vi "DetermineStateOfBoat-OLD.vi"() -> (2 "TimeSpentInCurrentState (s)":dbl, 3 "StateOfBoat":T1)   [LabVIEW 2013]
doc: "Eric Schneider and Bonnie Ishiguro\n1/24/14\n\nDetermineStateOfBoat should take in data from the forebrain about the plan of the boat (tacking, jibing, straight, distance to waypoint) as well as robot variables (heading, desired heading, wind speed, etc.) and makes a judgement about the qualitative state of the boat.\n\nThese qualitative states are intended to represent several different rules of sail/rudder control - which rules the sail/rudder should follow should change in each state. The set of current states is by no means set in stone, but should be tweaked with sailing advice so that in the end we have a handful of sailing states that each has a different control scheme for sail/rudder."
uses:
  Data/TypeDefs/Sailing State of Boat.ctl
panel:
  in  "Forebrain Maneuver\nCommand (PLACEHOLDER)":enum16{"No Maneuver", "Tack Now", "Jibe Now"}(ring)
  in  "MaxStayForce":dbl
  in  "WindSpeed (m/s)":dbl
  in  "HindbrainEmergencySailOverrideOn":bool
  in  "BoatSpeed (m/s)":dbl
  in  "RelativeWind (0-180)":dbl
  in  "DesiredHeading (0-360)":dbl
  in  "RobotHeading (0-360)":dbl
  in  "DistanceToNextWaypoint (m)":dbl=10.0
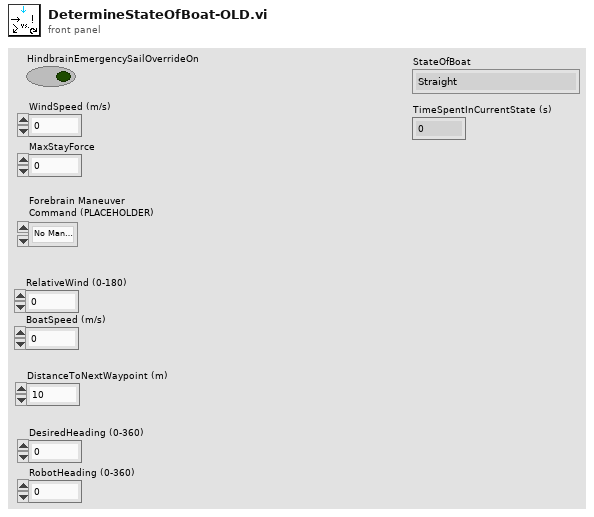
[diagram p1: front panel]
types:
  T1 = typedef "Sailing State of Boat.ctl" = enum16{"Straight", "Turning", "Approach Maneuver", "Cross Wind (Tack)", "Cross Wind (Jibe)", "Stuck in irons", "Turtle Mode"}
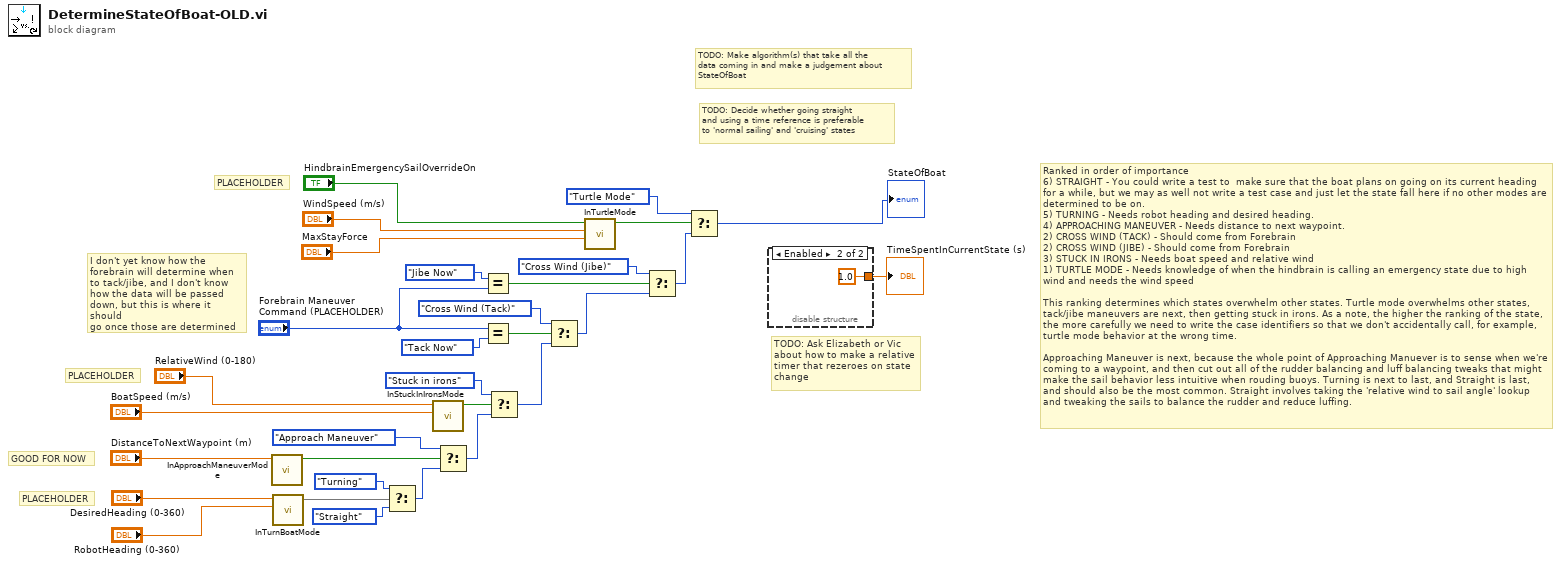
[diagram p0: block diagram]
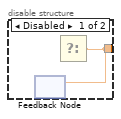
[diagram p2: hidden frame]
diagram:
  # "PLACEHOLDER"
  # "PLACEHOLDER"
  # "GOOD FOR NOW"
  # "PLACEHOLDER"
  # "I don't yet know how the\nforebrain will determine when\nto tack/jibe, and I don't know\nhow the data will be passed\ndown, but this is where it should\ngo once those are determined"
  # "Ranked in order of importance\n6) STRAIGHT - You could write a test to  make sure that the boat plans on going on its current heading for a while, but we may as well not write a test case and just let the state fall here if no other modes are determined to be on.\n5) TURNING - Needs robot heading and desired heading.\n4) APPROACHING MANEUVER - Needs distance to next waypoint.\n2) CROSS WIND (TACK) - Should come from Forebrain\n2) CROSS WIND (JIBE) - Should come from Forebrain\n3) STUCK IN IRONS - Needs boat speed and relative wind\n1) TURTLE MODE - Needs knowledge of when the hindbrain is calling an emergency state due to high wind and needs the wind speed\n\nThis ranking determines which states overwhelm other states. Turtle mode overwhelms other states, tack/jibe maneuvers are next, then getting stuck in irons. As a note, the higher the ranking of the state, the more carefully we need to write the case identifiers so that we don't accidentally call, for example, turtle mode behavior at the wrong time.\n\nApproaching Maneuver is next, because the whole point of Approaching Manuever is to sense when we're coming to a waypoint, and then cut out all of the rudder balancing and luff balancing tweaks that might make the sail behavior less intuitive when rouding buoys. Turning is next to last, and Straight is last, and should also be the most common. Straight involves taking the 'relative wind to sail angle' lookup and tweaking the sails to balance the rudder and reduce luffing."
  # "TODO: Ask Elizabeth or Vic about how to make a relative timer that rezeroes on state change"
  # "TODO: Decide whether going straight\nand using a time reference is preferable\nto 'normal sailing' and 'cruising' states"
  # "TODO: Make algorithm(s) that take all the\ndata coming in and make a judgement about\nStateOfBoat"
  n1 = call "InApproachManeuverMode.vi"("DistanceToNextWaypoint (m)"="DistanceToNextWaypoint (m)") -> ("InApproachManeuverMode?"=w22:bool)  [unwired: 10 in]
  n2 = call "InTurnBoatMode.vi"(10:"RobotHeading (0-360)", 11:"DesiredHeading (0-360)") -> (3:w27)  [unwired: 9 in]
  n3 = Select(t=Sailing_State_of_Boat."Turning", s=w27, f=Sailing_State_of_Boat."Straight" ("StateOfBoat")) -> (s? t:f=w29:T1)
  n4 = call "InStuckInIronsMode.vi"(10:"BoatSpeed (m/s)", "RelativeWind (0-180)"="RelativeWind (0-180)") -> ("InStuckInIronsMode?"=w12:bool)  [unwired: 9 in]
  n5 = Select(t=Sailing_State_of_Boat."Approach Maneuver", s=w22, f=w29) -> (s? t:f=w13:T1)
  n6 = Equal?(x=enum16{"No Maneuver", "Tack Now", "Jibe Now"}."Jibe Now" ("y"), y="Forebrain Maneuver\nCommand (PLACEHOLDER)") -> (x = y?=w17:bool)
  n7 = Equal?(x="Forebrain Maneuver\nCommand (PLACEHOLDER)", y=enum16{"No Maneuver", "Tack Now", "Jibe Now"}."Tack Now") -> (x = y?=w18:bool)
  n8 = Select(t=Sailing_State_of_Boat."Stuck in irons", s=w12, f=w13) -> (s? t:f=w8:T1)
  n9 = Select(t=Sailing_State_of_Boat."Cross Wind (Tack)", s=w18, f=w8) -> (s? t:f=w28:T1)
  n10 = call "InTurtleMode.vi"("MaxStayForce"="MaxStayForce", "WindSpeed (m/s)"="WindSpeed (m/s)", "HindbrainEmergencySailOverrideOn"="HindbrainEmergencySailOverrideOn") -> ("InTurtleMode?"=w5:bool)  [unwired: 8 in]
  n11 = Select(t=Sailing_State_of_Boat."Cross Wind (Jibe)", s=w17, f=w28) -> (s? t:f=w6:T1)
  n12 = Select(t=Sailing_State_of_Boat."Turtle Mode", s=w5, f=w6) -> (s? t:f=→"StateOfBoat":T1)
  n13 = disable-structure shown="Enabled" {
    disable-tunnel: [w32 1.0 ("TimeSpentInCurrentState")] -> w31
    frame Disabled {
      n14 = feedback #1() -> ()  [unwired: 2 in]
      n15 = Select() -> (s? t:f=w32:dbl)  [unwired: 3 in]
      n16 = feedback-in #1(w32) -> ()
    }
    frame Enabled {
    }
  }
  "TimeSpentInCurrentState (s)" <- w31
